vi "LassoLarsIC.vi"(8 "error in":errorcluster) -> (0 "error out":errorcluster, 3 "out":refnum<class "LassoLarsIC.lvclass">)   [LabVIEW 2020]
doc: "Lasso model fit with Lars using BIC or AIC for model selection\n\n The optimization objective for Lasso is::\n\n (1 / (2 * n_samples)) * ||y - Xw||^2_2 + alpha * ||w||_1\n\n AIC is the Akaike information criterion and BIC is the Bayes\n Information criterion. Such criteria are useful to select the value\n of the regularization parameter by making a trade-off between the\n goodness of fit and the complexity of the model. A good model should\n explain well the data while being simple.\n\n Read more in the :ref:`User Guide <least_angle_regression>`.\n\n Parameters\n ----------\n criterion : {'bic' , 'aic'}, default='aic'\n The type of criterion to use.\n\n fit_intercept : bool, default=True\n whether to calculate the intercept for this model. If set\n to false, no intercept will be used in calculations\n (i.e. data is expected to be centered).\n\n verbose : bool or int, default=False\n Sets the verbosity amount.\n\n normalize : bool, default=True\n This parameter is ignored when ``fit_intercept`` is set to False.\n If True, the regressors X will be normalized before regression by\n subtracting the mean and dividing by the l2-norm.\n If you wish to standardize, please use\n :class:`~sklearn.preprocessing.StandardScaler` before calling ``fit``\n on an estimator with ``normalize=False``.\n\n precompute : bool, 'auto' or array-like, default='auto'\n Whether to use a precomputed Gram matrix to speed up\n calculations. If set to ``'auto'`` let us decide. The Gram\n matrix can also be passed as argument.\n\n max_iter : int, default=500\n Maximum number of iterations to perform. Can be used for\n early stopping.\n\n eps : float, default=np.finfo(float).eps\n The machine-precision regularization in the computation of the\n Cholesky diagonal factors. Increase this for very ill-conditioned\n systems. Unlike the ``tol`` parameter in some iterative\n optimization-based algorithms, this parameter does not control\n the tolerance of the optimization.\n\n copy_X : bool, default=True\n If True, X will be copied; else, it may be overwritten.\n\n positive : bool, default=False\n Restrict coefficients to be >= 0. Be aware that you might want to\n remove fit_intercept which is set True by default.\n Under the positive restriction the model coefficients do not converge\n to the ordinary-least-squares solution for small values of alpha.\n Only coefficients up to the smallest alpha value (``alphas_[alphas_ >\n 0.].min()`` when fit_path=True) reached by the stepwise Lars-Lasso\n algorithm are typically in congruence with the solution of the\n coordinate descent Lasso estimator.\n As a consequence using LassoLarsIC only makes sense for problems where\n a sparse solution is expected and/or reached.\n\n Attributes\n ----------\n coef_ : array-like of shape (n_features,)\n parameter vector (w in the formulation formula)\n\n intercept_ : float\n independent term in decision function.\n\n alpha_ : float\n the alpha parameter chosen by the information criterion\n\n alphas_ : array-like of shape (n_alphas + 1,) or list of such arrays\n Maximum of covariances (in absolute value) at each iteration.\n ``n_alphas`` is either ``max_iter``, ``n_features`` or the\n number of nodes in the path with ``alpha >= alpha_min``, whichever\n is smaller. If a list, it will be of length `n_targets`.\n\n n_iter_ : int\n number of iterations run by lars_path to find the grid of\n alphas.\n\n criterion_ : array-like of shape (n_alphas,)\n The value of the information criteria ('aic', 'bic') across all\n alphas. The alpha which has the smallest information criterion is\n chosen. This value is larger by a factor of ``n_samples`` compared to\n Eqns. 2.15 and 2.16 in (Zou et al, 2007).\n\n\n \nAvailable methods:\nGet Attributes\nGet Params\nSet Params"
uses:
  LassoLarsIC.lvclass
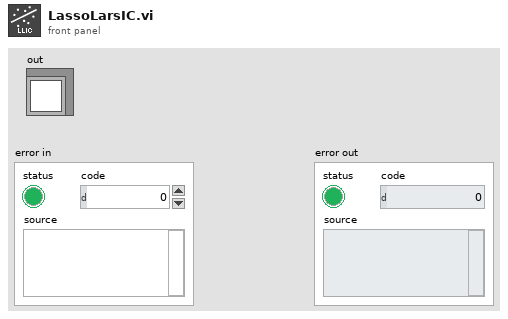
[diagram p1: front panel]
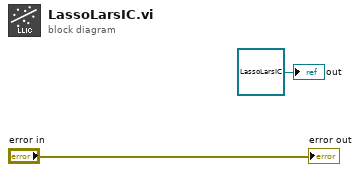
[diagram p0: block diagram]
diagram:
  "out" <- refnum<class "LassoLarsIC.lvclass"> refnum ("model")
  "error out" <- "error in"
